vi "K_S30_VISA F73.vi"(4 "error in":errorcluster, 6 "Channel":enum16{"CH0", "P1", "P2", "T", "TOB1", "TOB2"}(ring), 7 "Address":u8=250) -> (0 "error out":errorcluster, 2 "Status":u8 format="%.0b", 3 "Value":sgl format="%.6e")   [LabVIEW 2012]
panel:
  # "Function 73: Read Value of a Channel\nV1.0, b.v."
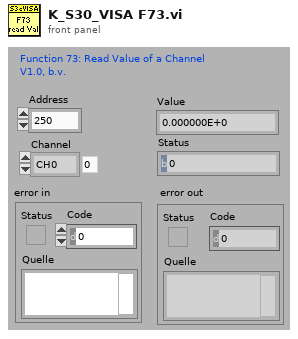
[diagram p1: front panel]
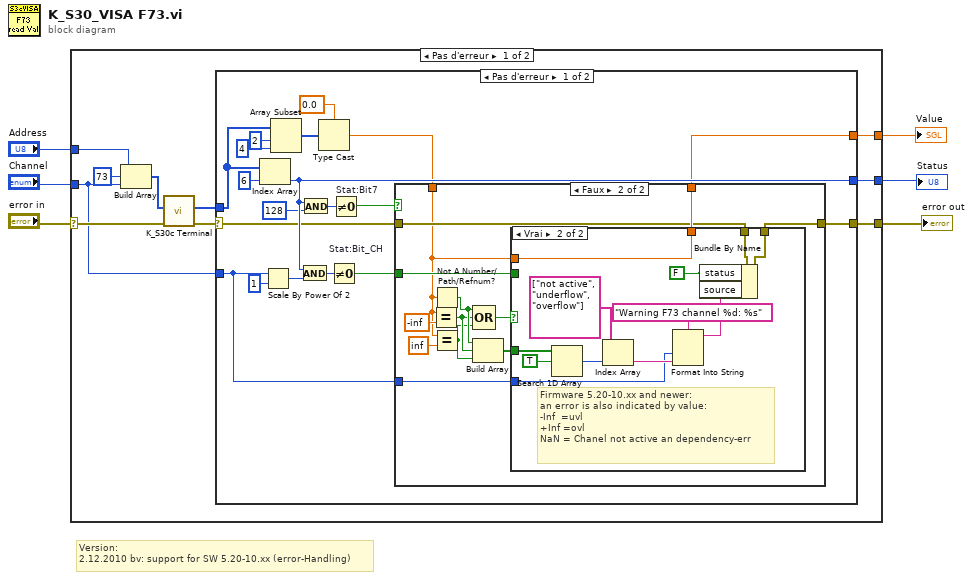
[diagram p0: block diagram]
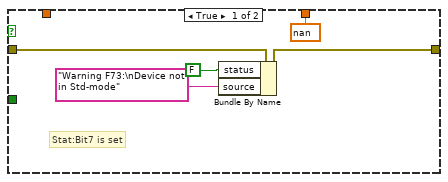
[diagram p2: hidden frame]
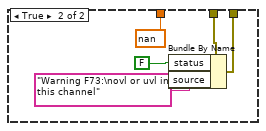
[diagram p4: hidden frame]
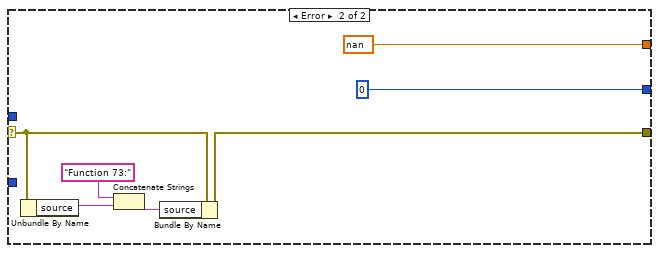
[diagram p5: hidden frame]
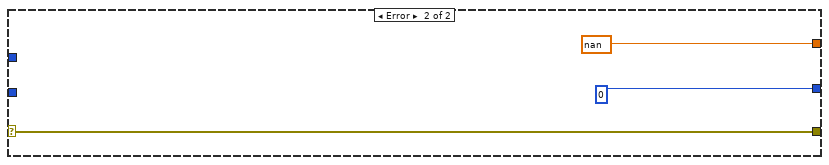
[diagram p6: hidden frame]
diagram:
  # "Version:\n2.12.2010 bv: support for SW 5.20-10.xx (error-Handling)"
  n1 = case shown="Pas d'erreur" "error in" {
    selector: "error in" -> [w13 w87]
    tunnel: "Address" -> [w16 _]
    tunnel: [w11 w87] -> w4
    tunnel: "Channel" -> [w9 _]
    tunnel: [w8 u8 0] -> w2
    tunnel: [w7 sgl nan] -> w1
    frame No Error {
      n2 = Build Array(w16, u8 73 ("Element"), w9) -> (w14:u16[])
      n3 = call "K_S30c Terminal.vi"("error in"=w13, "request"=w14) -> ("error out"=w12:errorcluster, "response"=w10:u8[])  [unwired: 4 in]
      n4 = case shown="Pas d'erreur" w12 {
        selector: w12 -> [w25 w84]
        tunnel: [w24 w82] -> w11
        tunnel: w10 -> [w31 _]
        tunnel: [w21 sgl nan] -> w7
        tunnel: [w28 u8 0] -> w8
        tunnel: w9 -> [w17 _]
        frame No Error {
          n5 = Index Array(array=w31, index=6 ("Index")) -> (element=w28:u8)
          n6 = Scale By Power Of 2(n=w17, x=u8 1) -> (x*2^n=w26:u8)
          n7 = Array Subset(array=w31, index=2 ("Index"), length=4 ("Länge")) -> (w32:u8[])
          n8 = And(x=w28, y=w26) -> (x .and. y?=w23:u8)
          n9 = And(x=w28, y=u8 128) -> (x .and. y?=w20:u8)
          n10 = Type Cast(type=sgl 0.0, x=w32) -> (*(type *) &x=w22:sgl)
          n11 = Not Equal To 0? "Stat:Bit_CH"(x=w23) -> (x != 0?=w18:bool)
          n12 = Not Equal To 0? "Stat:Bit7"(x=w20) -> (x != 0?=w19:bool)
          n13 = case shown="Faux" w19 {
            tunnel: w25 -> [w37 w48]
            tunnel: [w36 w47] -> w24
            tunnel: w22 -> [_ w42]
            tunnel: [sgl nan w50] -> w21
            tunnel: w18 -> [_ w49]
            tunnel: w17 -> [_ w41]
            frame True {
              # "Stat:Bit7 is set"
              n14 = Bundle By Name(cluster=w37, "status"=FALSE, "source"="Warning F73:\nDevice not in Std-mode") -> (w36:errorcluster)
            }
            frame False {
              n15 = Equal?(x=w42, y=sgl -inf) -> (x = y?=w45:bool)
              n16 = Not A Number/Path/Refnum?(number/path/refnum=w42) -> (NaN/Path/Refnum?=w46:bool)
              n17 = Equal?(x=w42, y=sgl inf) -> (x = y?=w44:bool)
              n18 = Compound Arithmetic op=OR(w46, w45, w44) -> (w51:bool)
              n19 = Build Array(w46, w45, w44) -> (w43:bool[])
              n20 = case shown="Vrai" w51 {
                tunnel: w42 -> [w56 w77]
                tunnel: [w58 w77] -> w50
                tunnel: w49 -> [w57 _]
                tunnel: w48 -> [w55 w74]
                tunnel: [w54 w75] -> w47
                tunnel: w43 -> [_ w73]
                tunnel: w41 -> [_ w67]
                frame False {
                  # "Check status-Byte for the actual Channel:\nFor SW-Version before 5.20-10.xx"
                  n21 = case shown="Faux" w57 {
                    tunnel: [w60 sgl nan] -> w58
                    tunnel: w56 -> [w60 _]
                    tunnel: w55 -> [w59 w62]
                    tunnel: [w59 w61] -> w54
                    frame False {
                    }
                    frame True {
                      n22 = Bundle By Name(cluster=w62, "status"=FALSE, "source"="Warning F73:\novl or uvl in this channel") -> (w61:errorcluster)
                    }
                  }
                }
                frame True {
                  # "Firmware 5.20-10.xx and newer:\nan error is also indicated by value: \n-Inf  =uvl\n+Inf =ovl\nNaN = Chanel not active an dependency-err"
                  n23 = Search 1D Array(1D array=w73, element=TRUE ("Element")) -> (index of element=w71:i32)  [unwired: 1 in]
                  n24 = Index Array(array=string[] ["not active", "underflow", "overflow"], index=w71) -> (element=w68:string)
                  n25 = Format Into String(format string="Warning F73 channel %d: %s", w67, w68) -> (resulting string=w66:string)  [unwired: 2 in, 1 out]
                  n26 = Bundle By Name(cluster=w74, "status"=FALSE, "source"=w66) -> (w75:errorcluster)
                }
              }
            }
          }
        }
        frame Error {
          n27 = Unbundle By Name(w84) -> ("source"=w80:string)
          n28 = Concatenate Strings("Function 73:" ("String"), w80) -> (w83:string)
          n29 = Bundle By Name(cluster=w84, "source"=w83) -> (w82:errorcluster)
        }
      }
    }
    frame Error {
    }
  }
  "error out" <- w4
  "Status" <- w2
  "Value" <- w1
